vi "Swerve Controller.vi"(8 "error in":errorcluster) -> ()   [LabVIEW 2020]
doc: "This VI executes continuously carrying out the current operation and responding to updates or new operations. It will often contain the timing or control code that is difficult to place directly in TeleOp. This VI generally opens all sensors and motors and isolates the rest of the robot code from knowing how the operations are carried out."
uses:
  <vilib>/Rock Robotics/WPI/Framework/Completion Status.ctl
  Swerve Setpoints.ctl
  Swerve Operations.ctl
  <vilib>/addons/control/pid/pid.llb/PID (DBL).vi
  <vilib>/addons/control/pid/NI_PID_pid.lvlib
  <vilib>/Rock Robotics/Network Tables/NT Write Boolean.vi
panel:
  in  "PID gains 2":T1={"proportional gain (Kc)"=1.0, "integral time (Ti, min)"=0.01, "derivative time (Td, min)"=0.0} {"derivative time (Td, min)" format="%.3f"; "integral time (Ti, min)" format="%.3f"; "proportional gain (Kc)" format="%.3f"}
  in  "PID gains":T1={"proportional gain (Kc)"=1.0, "integral time (Ti, min)"=0.01, "derivative time (Td, min)"=0.0} {"derivative time (Td, min)" format="%.3f"; "integral time (Ti, min)" format="%.3f"; "proportional gain (Kc)" format="%.3f"}
  in  "Interactive Values":T2
  out "Current\nCmd":string
  in  "Buttons":cluster{"Execute Cmd":bool, "Abort Cmd":bool}
  out "Command Timing":cluster{"Start Time (ms)":u32, "Iterations":i32}
  out "Status":T4
  # "Tip: It may be helpful to observe inputs and sensor values.\nYou may also want to display tuning or debugging controls."
  # "Interactive Command: You may fill in the settings for a command\nand schedule it with the Execute button. You can observe and abort\nany command while fine tuning the code for the controller."
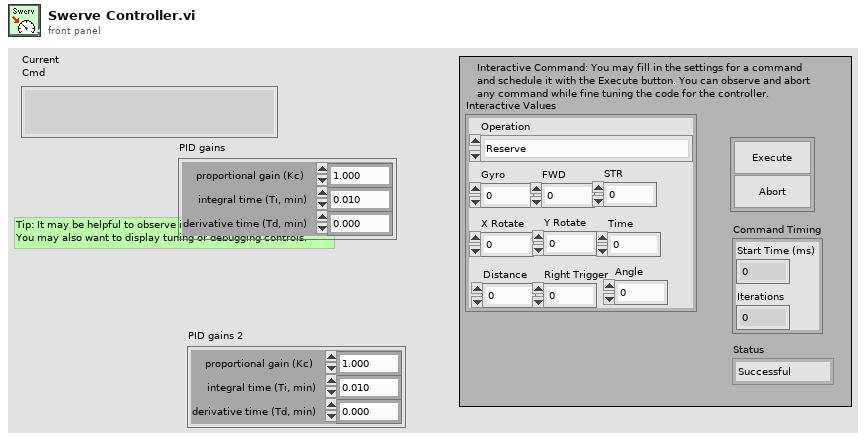
[diagram p1: front panel]
types:
  T1 = cluster{"proportional gain (Kc)":dbl, "integral time (Ti, min)":dbl, "derivative time (Td, min)":dbl}
  T2 = typedef "Swerve Setpoints.ctl" = cluster{"Operation":T3, "Gyro":dbl, "X Rotate":dbl, "FWD":dbl, "STR":dbl, "Time":dbl, "Angle":dbl, "Distance":dbl, "Right Trigger":dbl, "Y Rotate":dbl}
  T3 = typedef "Swerve Operations.ctl" = enum16{"Reserve", "Read Current", "Immediate", "Joystick Drive", "Drive for Distance", "Drive for Time", "Turn to Angle", "Drive to Angle(Time)", "Drive to Angle(Distance)"}
  T4 = typedef "Completion Status.ctl" = enum16{"Successful", "Aborted", "Incomplete"}
  T5 = typedef "Command Status Info.ctl" = cluster{"Name":string, "Status":T4, "notifier out":T6}
  T6 = typedef "Completion Notifier.ctl" = refnum<notifier>
  T7 = cluster{"Current Command":T2, "Command Timing":cluster{"Start Time (ms)":u32, "Iterations":i32}, "Command Arguments":cluster{"Command Info":T5, "Description":string, "Default Command":T2, "queue out":refnum<queue>, "Subsystem Name":string}}
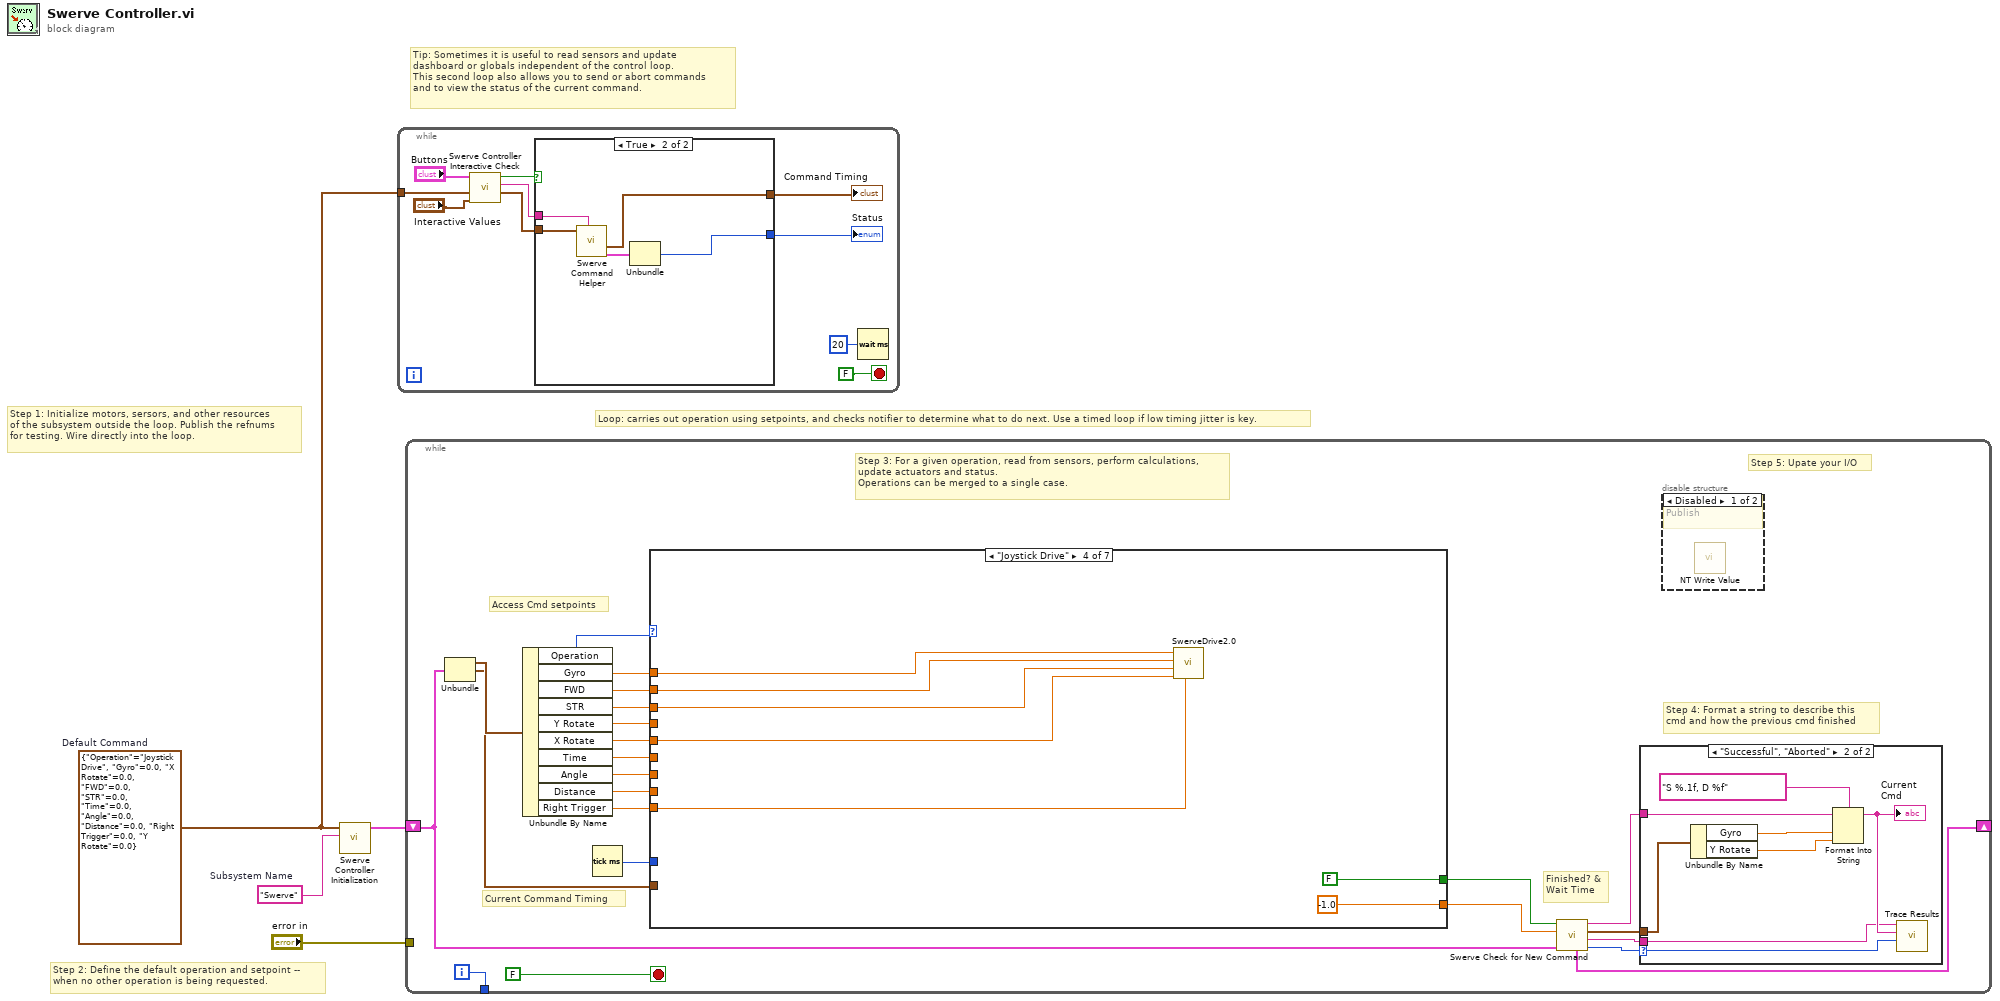
[diagram p0: block diagram]
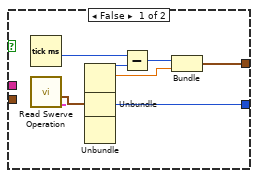
[diagram p2: hidden frame]
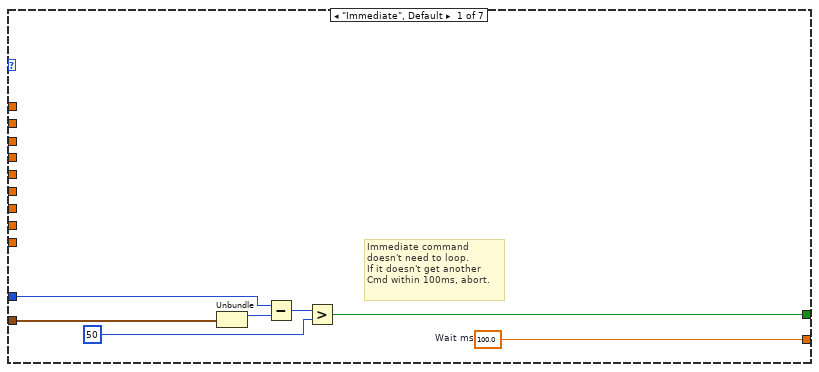
[diagram p5: hidden frame]
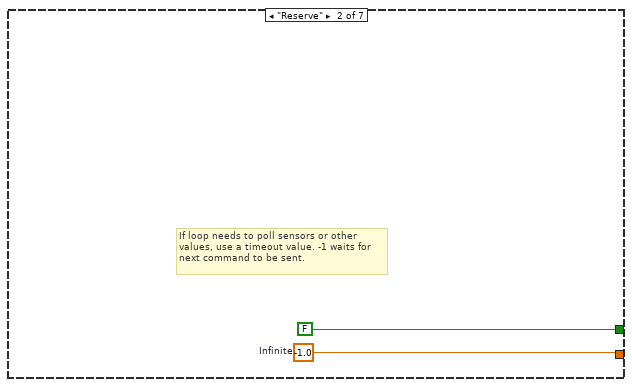
[diagram p6: hidden frame]
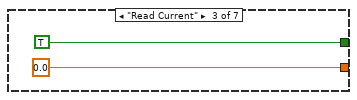
[diagram p7: hidden frame]
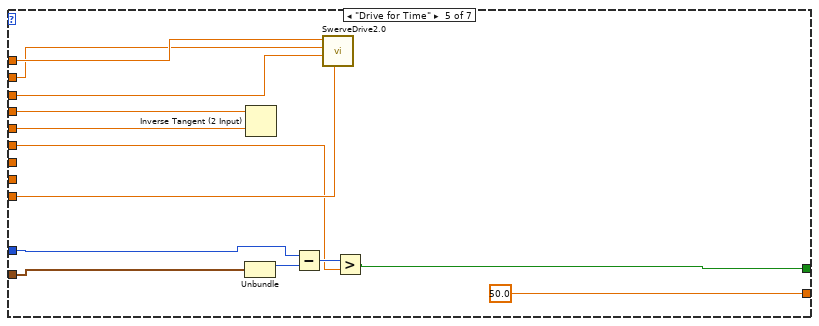
[diagram p8: hidden frame]
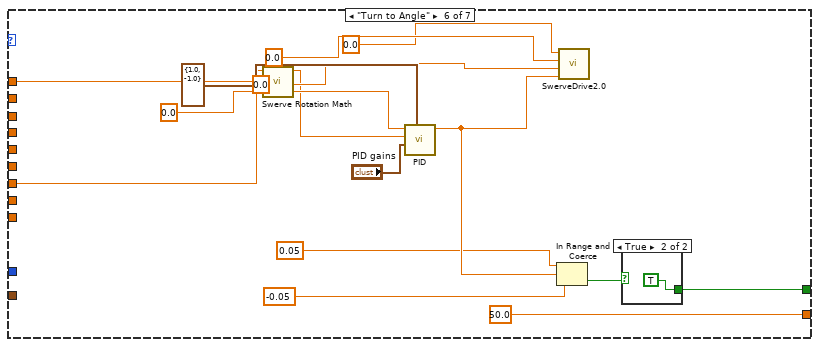
[diagram p9: hidden frame]
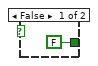
[diagram p10: hidden frame]
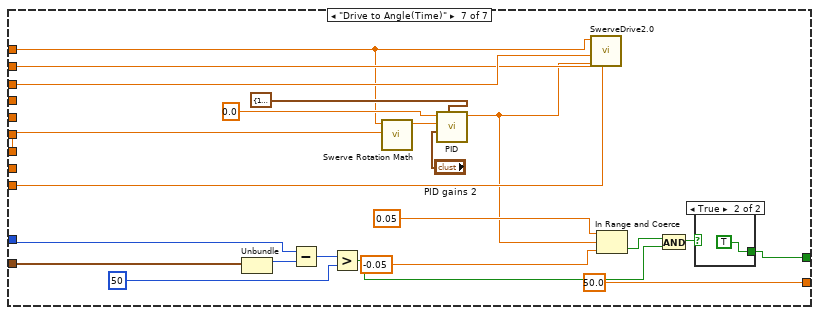
[diagram p11: hidden frame]
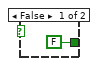
[diagram p12: hidden frame]
diagram:
  w1 = T2 {"Operation"=enum."Joystick Drive", "Gyro"=0.0, "X Rotate"=0.0, "FWD"=0.0, "STR"=0.0, "Time"=0.0, "Angle"=0.0, "Distance"=0.0, "Right Trigger"=0.0, "Y Rotate"=0.0}  # Default Command
  w2 = "Swerve"  # Subsystem Name
  # "Tip: Sometimes it is useful to read sensors and update\ndashboard or globals independent of the control loop.\nThis second loop also allows you to send or abort commands\nand to view the status of the current command."
  # "Step 2: Define the default operation and setpoint --\nwhen no other operation is being requested."
  # "Step 1: Initialize motors, sersors, and other resources\nof the subsystem outside the loop. Publish the refnums\nfor testing. Wire directly into the loop."
  # "Loop: carries out operation using setpoints, and checks notifier to determine what to do next. Use a timed loop if low timing jitter is key."
  n1 = call "Swerve Controller Initialization.vi"("Subsystem Name"=w2, "Default Command"=w1) -> ("Current Command"=w3:T7)  [unwired: 9 in]
  n2 = while {
    tunnel: w1 -> [w11]
    stop <- FALSE stop-if-true
    n3 = call "Swerve Controller Interactive Check.vi"("Interactive Command in"="Interactive Values", "Default Command"=w11, "Buttons"="Buttons") -> ("Interactive Command out"=w8:T2, "Trace String"=w9:string, "Schedule"=w10:bool)  [unwired: 6 in]
    n4 = case shown="True" w10 {
      tunnel: [w22 w27] -> w7
      tunnel: w8 -> [_ w25]
      tunnel: [w18 w23] -> w6
      tunnel: w9 -> [_ w26]
      frame False {
        n5 = Tick Count (ms)() -> (millisecond timer value=w17:u32)
        n6 = call "Read Swerve Operation.vi"() -> ("Command Info"=w15:T5, "SubSystem Data"=w16:T2)  [unwired: 9 in, 1 out]
        n7 = Unbundle(w16) -> ("Operation"=w21:T3, "Gyro"=w19:dbl)  [unwired: 8 out]
        n8 = Unbundle(w15) -> ("Status"=w22:T4)  [unwired: 2 out]
        n9 = Subtract(x=w17, y=w21) -> (x-y=w20:u32)
        n10 = Bundle(w20, "Gyro"=w19) -> (w18:cluster{u32, "Gyro":dbl})  [unwired: 1 in]
      }
      frame True {
        n11 = call "Swerve Command Helper.vi"("Description"=w26, "SubSystem Data"=w25) -> ("Command Info Out"=w24:T5, "Command Timing"=w23:cluster{"Start Time (ms)":u32, "Iterations":i32})  [unwired: 7 in, 1 out]
        n12 = Unbundle(w24) -> ("Status"=w27:T4)  [unwired: 2 out]
      }
    }
    "Status" <- w7
    "Command Timing" <- w6
    n13 = Wait (ms)(milliseconds to wait=u32 20) -> ()  [unwired: 1 out]
  }
  n14 = while {
    shift-right: [w44] -> _
    shift-left: w3 -> [w37]
    tunnel: [w49] -> _
    tunnel: "error in" -> [_]
    i -> [w49]
    stop <- FALSE stop-if-true
    # "Step 5: Upate your I/O"
    # "Step 4: Format a string to describe this\ncmd and how the previous cmd finished"
    # "Current Command Timing"
    # "Access Cmd setpoints"
    # "Finished? &\nWait Time"
    # "Step 3: For a given operation, read from sensors, perform calculations,\nupdate actuators and status.\nOperations can be merged to a single case."
    n15 = Unbundle(w37) -> ("Current Command"=w48:T2, "Command Timing"=w45:cluster{"Start Time (ms)":u32, "Iterations":i32})  [unwired: 1 out]
    n16 = Unbundle By Name(w48) -> ("Operation"=w47:T3, "Gyro"=w36:dbl, "FWD"=w35:dbl, "STR"=w34:dbl, "Y Rotate"=w33:dbl, "X Rotate"=w28:dbl, "Time"=w29:dbl, "Angle"=w32:dbl, "Distance"=w31:dbl, "Right Trigger"=w30:dbl)
    n17 = Tick Count (ms)() -> (millisecond timer value=w46:u32)
    n18 = case shown="\"Joystick Drive\"" w47 {
      tunnel: [w65 w67 0.0 ("Time") -1.0 ("Infinite") 50.0 ("Time") 50.0 ("Time") 50.0 ("Time")] -> w42
      tunnel: [w59 FALSE ("ignore previous (F)") TRUE ("ignore previous (F)") FALSE ("ignore previous (F)") w81 w95 w117] -> w43
      tunnel: w45 -> [w61 _ _ _ w82 _ w112]
      tunnel: w46 -> [w60 _ _ _ w83 _ w111]
      tunnel: w36 -> [_ _ _ w72 w89 w98 w121]
      tunnel: w35 -> [_ _ _ w76 w86 _ w122]
      tunnel: w34 -> [_ _ _ w70 w87 _ w123]
      tunnel: w33 -> [_ _ _ _ w77 _ _]
      tunnel: w32 -> [_ _ _ _ _ w97 w120]
      tunnel: w31 -> [_ _ _ _ _ _ _]
      tunnel: w30 -> [_ _ _ w75 w88 _ w124]
      tunnel: w29 -> [_ _ _ _ w79 _ _]
      tunnel: w28 -> [_ _ _ w71 w78 _ _]
      frame "Immediate", Default {
        w65 = 100.0  # Wait ms
        # "Immediate command\ndoesn't need to loop.\nIf it doesn't get another\nCmd within 100ms, abort."
        n19 = Unbundle(w61) -> ("Start Time (ms)"=w64:u32)  [unwired: 1 out]
        n20 = Subtract(x=w60, y=w64) -> (x-y=w63:u32)
        n21 = Greater?(x=w63, y=u8 50 ("Left Motor")) -> (0:w59:bool)
      }
      frame "Reserve" {
        w67 = -1.0  # Infinite
        # "If loop needs to poll sensors or other\nvalues, use a timeout value. -1 waits for\nnext command to be sent."
      }
      frame "Read Current" {
      }
      frame "Joystick Drive" {
        n22 = call "SwerveDrive2.0.vi"("Right Trigger"=w75, "RCW"=w71, "STR"=w70, "FWD"=w76, "Gyro"=w72) -> ()  [unwired: 7 in]
      }
      frame "Drive for Time" {
        n23 = Unbundle(w82) -> ("Start Time (ms)"=w85:u32)  [unwired: 1 out]
        n24 = Inverse Tangent (2 Input)(1:w78, 2:w77) -> ()  [unwired: 1 out]
        n25 = Subtract(x=w83, y=w85) -> (x-y=w84:u32)
        n26 = call "SwerveDrive2.0.vi"("Right Trigger"=w88, "STR"=w87, "FWD"=w86, "Gyro"=w89) -> ()  [unwired: 8 in]
        n27 = Greater?(x=w84, y=w79) -> (0:w81:bool)
      }
      frame "Turn to Angle" {
        n28 = call "Swerve Rotation Math.vi"("Wheel Angle"=w97, "Encoder"=w98) -> ("Difference"=w96:dbl)  [unwired: 7 in, 2 out]
        n29 = call-poly <vilib>:"PID.vi"("output range"=cluster{"output high":dbl, "output low":dbl} {"output high"=1.0, "output low"=-1.0}, "PID gains"="PID gains", "process variable"=w96, "setpoint"=0.0) -> ("output"=w93:dbl)  [unwired: 6 in, 1 out]
        n30 = In Range and Coerce(upper limit=0.05, x=w93, lower limit=-0.05) -> (In Range?=w94:bool)  [unwired: 1 out]
        n31 = call "SwerveDrive2.0.vi"("RCW"=w93, "STR"=0.0, "FWD"=0.0, "Gyro"=0.0) -> ()  [unwired: 8 in]
        n32 = case shown="True" w94 {
          tunnel: [FALSE ("ignore previous (F)") TRUE ("ignore previous (F)")] -> w95
          frame False {
          }
          frame True {
          }
        }
      }
      frame "Drive to Angle(Time)" {
        n33 = Unbundle(w112) -> ("Start Time (ms)"=w115:u32)  [unwired: 1 out]
        n34 = Subtract(x=w111, y=w115) -> (x-y=w114:u32)
        n35 = Greater?(x=w114, y=u8 50 ("Left Motor")) -> (0:w108:bool)
        n36 = call "Swerve Rotation Math.vi"("Wheel Angle"=w120, "Encoder"=w121) -> ("Difference"=w125:dbl)  [unwired: 7 in, 2 out]
        n37 = call-poly <vilib>:"PID.vi"("output range"=cluster{"output high":dbl, "output low":dbl} {"output high"=1.0, "output low"=-1.0}, "PID gains"="PID gains 2", "process variable"=w125, "setpoint"=0.0) -> ("output"=w116:dbl)  [unwired: 6 in, 1 out]
        n38 = call "SwerveDrive2.0.vi"("Right Trigger"=w124, "RCW"=w116, "STR"=w123, "FWD"=w122, "Gyro"=w121) -> ()  [unwired: 7 in]
        n39 = In Range and Coerce(upper limit=0.05, x=w116, lower limit=-0.05) -> (In Range?=w109:bool)  [unwired: 1 out]
        n40 = And(x=w109, y=w108) -> (x .and. y?=w110:bool)
        n41 = case shown="True" w110 {
          tunnel: [FALSE ("ignore previous (F)") TRUE ("ignore previous (F)")] -> w117
          frame False {
          }
          frame True {
          }
        }
      }
    }
    n42 = call "Swerve Check for New Command.vi"("Current Command"=w37, "Wait time (ms)"=w42, "Finished?"=w43) -> ("Completion"=w38:T4, "Subsystem Name"=w39:string, "Current Command"=w40:T2, "Initial Trace String"=w41:string, "NextCommand"=w44:T7)  [unwired: 4 in]
    n43 = case shown="\"Successful\", \"Aborted\"" w38 {
      selector: w38 -> [_ w58]
      tunnel: w41 -> [_ w54]
      tunnel: w40 -> [_ w55]
      tunnel: w39 -> [_ w51]
      frame "Incomplete", Default {
        # "Continuing current command"
      }
      frame "Successful", "Aborted" {
        # "Report and setup for next command"
        n44 = Unbundle By Name(w55) -> ("Gyro"=w57:dbl, "Y Rotate"=w52:dbl)
        n45 = Format Into String(format string="S %.1f, D %f", initial string=w54, w57, w52) -> (resulting string=w53:string)  [unwired: 1 in, 1 out]
        "Current\nCmd" <- w53
        n46 = call <vilib>:"Trace Results.vi"("Status of previous command"=w58, "Description"=w53, "Subsystem"=w51) -> ()  [unwired: 9 in]
      }
    }
    n47 = disable-structure shown="Disabled" {
      frame Disabled {
        # "Publish"
        n48 = call-poly <vilib>:"NT Write Value.vi"() -> ()  [unwired: 11 in, 1 out]
      }
      frame Enabled {
      }
    }
  }
